vi "AutoScreenShot.vi"(2 "Params Save":T2, 3 "Figure image data":T3, 4 "Datasetname":string) -> (1 "imagefilename":string)   [LabVIEW 2019]
doc: "Create image file with transparent name in CARODOC/attachments/%y-%m-%d"
uses:
  <vilib>/picture/picture.llb/imagedata.ctl
  TypeDefs/AcqMode.ctl
panel:
  out "Experiment Name":string
  out "created path":path
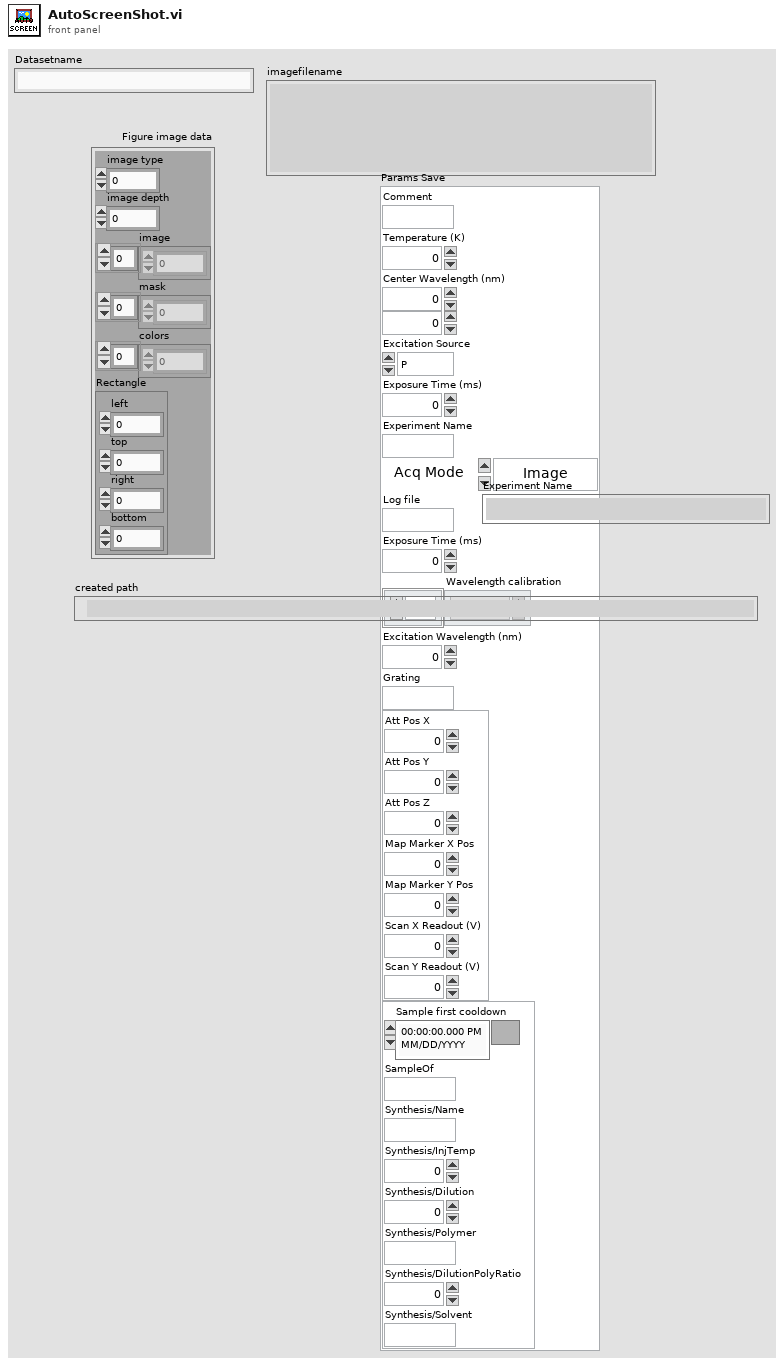
[diagram p1: front panel]
types:
  T1 = typedef "AcqMode.ctl" = enum16{"Image", "Spectrum", "APD 1", "APD 2", "APD 1+2"}
  T2 = cluster{"Comment":string, "Temperature (K)":dbl, "Center Wavelength (nm)":dbl, "Numeric":dbl, "Excitation Source":enum16{"P", "CW", "SK"}, "Exposure Time (ms)":dbl, "Experiment Name":string, "Acq Mode":T1, "Log file":string, "Exposure Time (ms)":dbl, "Wavelength calibration":dbl[], "Excitation Wavelength (nm)":dbl, "Grating":string, "Cluster":cluster{"Att Pos X":dbl, "Att Pos Y":dbl, "Att Pos Z":dbl, "Map Marker X Pos":i8, "Map Marker Y Pos":i8, "Scan X Readout (V)":dbl, "Scan Y Readout (V)":dbl}, "Cluster":cluster{"Sample first cooldown":timestamp, "SampleOf":string, "Synthesis/Name":string, "Synthesis/InjTemp":dbl, "Synthesis/Dilution":dbl, "Synthesis/Polymer":string, "Synthesis/DilutionPolyRatio":dbl, "Synthesis/Solvent":string}}
  T3 = typedef "imagedata.ctl" = cluster{"image type":i32, "image depth":i32, "image":u8[], "mask":u8[], "colors":u32[], "Rectangle":cluster{"left":i16, "top":i16, "right":i16, "bottom":i16}}
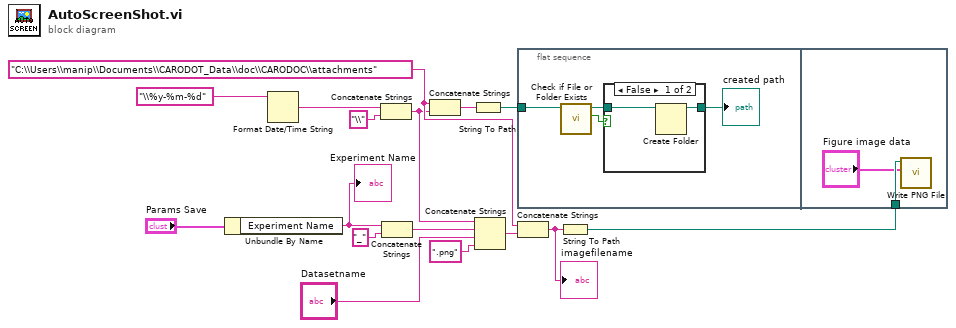
[diagram p0: block diagram]
diagram:
  w6 = "C:\\Users\\manip\\Documents\\CARODOT_Data\\doc\\CARODOC\\attachments"
  n1 = Unbundle By Name("Params Save") -> ("Experiment Name"=w8:string)
  "Experiment Name" <- w8
  n2 = Format Date/Time String(time format string (%c)="\\%y-%m-%d") -> (date/time string=w5:string)  [unwired: 2 in]
  n3 = Concatenate Strings(w5, "\\" ("string")) -> (w2:string)
  n4 = Concatenate Strings(w8, "_" ("string")) -> (w7:string)
  n5 = Concatenate Strings(w6, w2) -> (w4:string)
  n6 = String To Path(string=w4) -> (path=w3:path)
  n7 = Concatenate Strings(w2, w7, "Datasetname", ".png" ("string")) -> (w12:string)
  n8 = flat-sequence {
    tunnel: w3 -> [w19]
    tunnel: w1 -> [w25]
    frame #0 {
      n9 = call <vilib>:"Check if File or Folder Exists.vi"("path"=w19) -> ("file or folder exists?"=w18:bool, "dup path"=w17:path)  [unwired: 8 in, 1 out]
      n10 = case shown="False" w18 {
        tunnel: [w22 w23] -> w20
        tunnel: w17 -> [w21 w23]
        frame False {
          n11 = Create Folder(path (use dialog)=w21) -> (created path=w22:path)  [unwired: 2 in, 2 out]
        }
        frame True {
        }
      }
      "created path" <- w20
    }
    frame #1 {
      n12 = call <vilib>:"Write PNG File.vi"("image data"="Figure image data", "path to PNG file"=w25) -> ()  [unwired: 8 in, 2 out]
    }
  }
  n13 = Concatenate Strings(w6, w12) -> (w14:string)
  "imagefilename" <- w14
  n14 = String To Path(string=w14) -> (path=w1:path)
